vi "Do.vi"(8 "error in (no error)":errorcluster, 10 "Actor in":refnum<class "Actor.lvclass">, 11 "Update Write Ringdowns MSG":refnum<class "Update Write Ringdowns MSG.lvclass">) -> (0 "error out":errorcluster, 2 "Actor out":refnum<class "Actor.lvclass">)   [LabVIEW 2014, in "eCRDS Library.lvlib" / "Update Write Ringdowns MSG.lvclass"]
doc: "(<B>Filename</B>: Actor Framework.lvlib:Message.lvclass:Do.vi)\n\nDefines what a message does when it is received by an actor. Generally, a message instructs an actor to invoke one of its methods. By default, this method does nothing. A child class must override it to define behavior. Create a child class by using the Actor Framework Message Maker dialog box."
uses:
  Update Write Ringdowns MSG.lvclass
  <vilib>/ActorFramework/Actor/Actor.lvclass
  Update Write Ringdowns MSG.lvclass/Update Write Ringdowns MSG.ctl
  Instr Actor/Instr Actor.lvclass
  Commands/Write Ringdowns/Set Write Ringdowns CMD.lvclass
  Commands/Write Ringdowns/Set Write Ringdowns CMD.lvclass/Set Write Ringdowns CMD.ctl
  Commands/Write Ringdowns/Write write_.vi
  Instr Actor/Accessors/Read CMD.vi
  reusable/Command/Command.lvclass
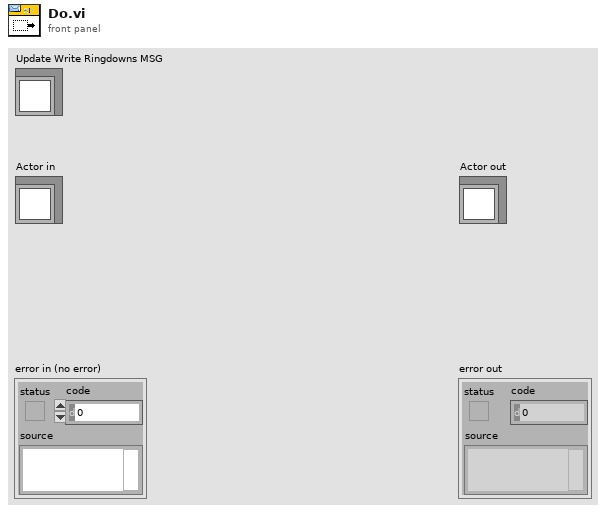
[diagram p1: front panel]
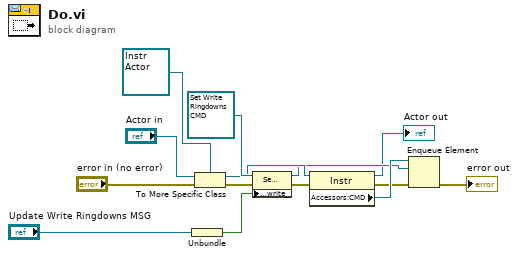
[diagram p0: block diagram]
diagram:
  n1 = Unbundle("Update Write Ringdowns MSG") -> (w10:bool)
  n2 = To More Specific Class(target class=refnum<class "Instr Actor.lvclass"> refnum ("Instrument Lib:Instr"), reference="Actor in", error in="error in (no error)") -> (specific class reference=w9:refnum<class "Instr Actor.lvclass">, error out=w4:errorcluster)
  n3 = property class="Set Write Ringdowns CMD"(reference=refnum<class "Set Write Ringdowns CMD.lvclass"> refnum ("eCRDS Library.lvlib:Set Write Ringdowns CMD"), error in=w4, "Accessors:write_"=w10) -> (reference out=w7:refnum<class "Set Write Ringdowns CMD.lvclass">, error out=w3:errorcluster)
  n4 = property class="Instr"(reference=w9, error in=w3) -> (reference out=→"Actor out":refnum<class "Instr Actor.lvclass">, error out=w2:errorcluster, "Accessors:CMD"=w8:refnum<queue>)
  n5 = Enqueue Element(queue=w8, element=w7, error in (no error)=w2) -> (error out=→"error out":errorcluster)  [unwired: 1 in, 2 out]
